vi "Holzworth.vi"(10 "Stop Point":string, 11 "Holzworth":refnum<visa-resource-name>="COM9") -> (2 "Amplitudes":string[](array[string]), 3 "Frequencies":string[](array[string]))   [LabVIEW 2023]
uses:
  <vilib>/regexp/Match Regular Expression.xnode
panel:
  out "read buffer 9":string
  out "read buffer 8":string
  out "read buffer 7":string
  out "read buffer 6":string
  out "read buffer 5":string
  out "read buffer 4":string
  out "read buffer 2":string
  out "points":dbl
  out "Comma Count":i32
  out "String 2":string
  out "String":string
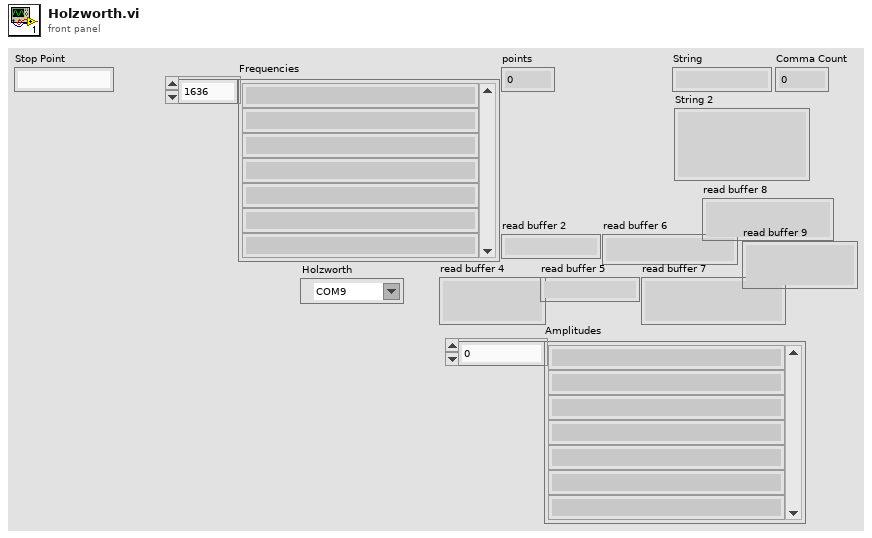
[diagram p1: front panel]
diagram:
  n1 = VISA Open(VISA resource name="Holzworth") -> (VISA resource name=w87:refnum<visa-resource-name>, error out=w84:errorcluster)  [unwired: 4 in]
  n2 = VISA Set I/O Buffer Size(VISA resource name=w87, size (4096)=u32 30000, error in (no error)=w84) -> (VISA resource name out=w86:refnum<visa-resource-name>, error out=w85:errorcluster)  [unwired: 1 in]
  n3 = VISA Flush I/O Buffer(VISA resource name=w86, error in (no error)=w85) -> (VISA resource name out=w4:refnum<visa-resource-name>, error out=w3:errorcluster)  [unwired: 1 in]
  n4 = Concatenate Strings("*RST" ("write buffer"), "\r") -> (w158:string)
  n5 = VISA Write(VISA resource name=w4, write buffer=w158, error in (no error)=w3) -> (VISA resource name out=w92:refnum<visa-resource-name>, error out=w90:errorcluster)  [unwired: 1 out]
  n6 = flat-sequence {
    tunnel: w92 -> [w163]
    tunnel: [w163] -> w91
    tunnel: w90 -> [w162]
    tunnel: [w162] -> w89
    tunnel: [w168] -> w48
    tunnel: [w169] -> w47
    tunnel: w91 -> [w167]
    tunnel: w89 -> [w166]
    frame #0 {
      n7 = Wait (ms)(milliseconds to wait=u32 2000) -> ()  [unwired: 1 out]
    }
    frame #1 {
      n8 = VISA Read(VISA resource name=w167, byte count=u32 256, error in (no error)=w166) -> (VISA resource name out=w168:refnum<visa-resource-name>, read buffer=→"read buffer 2":string, error out=w169:errorcluster)  [unwired: 1 out]
    }
  }
  n9 = Concatenate Strings(":SENS:PN:MEAS:TYPE:ABSOLUTE" ("write buffer"), "\r") -> (w58:string)
  n10 = VISA Write(VISA resource name=w48, write buffer=w58, error in (no error)=w47) -> (VISA resource name out=w60:refnum<visa-resource-name>, error out=w59:errorcluster)  [unwired: 1 out]
  n11 = flat-sequence {
    tunnel: w60 -> [w172]
    tunnel: [w172] -> w62
    tunnel: w59 -> [w171]
    tunnel: [w171] -> w61
    tunnel: [w177] -> w50
    tunnel: [w178] -> w49
    tunnel: w62 -> [w176]
    tunnel: w61 -> [w175]
    frame #0 {
      n12 = Wait (ms)(milliseconds to wait=u32 2000) -> ()  [unwired: 1 out]
    }
    frame #1 {
      n13 = VISA Read(VISA resource name=w176, byte count=u32 256, error in (no error)=w175) -> (VISA resource name out=w177:refnum<visa-resource-name>, read buffer=→"read buffer 4":string, error out=w178:errorcluster)  [unwired: 1 out]
    }
  }
  n14 = Concatenate Strings(":SENS:PN:MODE:SINGLE" ("write buffer"), "\r") -> (w51:string)
  n15 = VISA Write(VISA resource name=w50, write buffer=w51, error in (no error)=w49) -> (VISA resource name out=w53:refnum<visa-resource-name>, error out=w52:errorcluster)  [unwired: 1 out]
  n16 = flat-sequence {
    tunnel: w53 -> [w181]
    tunnel: [w181] -> w57
    tunnel: w52 -> [w180]
    tunnel: [w180] -> w56
    tunnel: [w187] -> w38
    tunnel: w57 -> [w186]
    tunnel: w56 -> [w185]
    tunnel: [w184] -> w39
    frame #0 {
      n17 = Wait (ms)(milliseconds to wait=u32 2000) -> ()  [unwired: 1 out]
    }
    frame #1 {
      n18 = VISA Read(VISA resource name=w186, byte count=u32 256, error in (no error)=w185) -> (VISA resource name out=w184:refnum<visa-resource-name>, read buffer=→"read buffer 5":string, error out=w187:errorcluster)  [unwired: 1 out]
    }
  }
  n19 = Concatenate Strings(":SENS:PN:CORR:COUN:1000" ("write buffer"), "\r") -> (w40:string)
  n20 = VISA Write(VISA resource name=w39, write buffer=w40, error in (no error)=w38) -> (VISA resource name out=w42:refnum<visa-resource-name>, error out=w41:errorcluster)  [unwired: 1 out]
  n21 = flat-sequence {
    tunnel: w42 -> [w190]
    tunnel: [w190] -> w44
    tunnel: w41 -> [w189]
    tunnel: [w189] -> w43
    tunnel: [w196] -> w29
    tunnel: w44 -> [w195]
    tunnel: w43 -> [w194]
    tunnel: [w193] -> w30
    frame #0 {
      n22 = Wait (ms)(milliseconds to wait=u32 2000) -> ()  [unwired: 1 out]
    }
    frame #1 {
      n23 = VISA Read(VISA resource name=w195, byte count=u32 256, error in (no error)=w194) -> (VISA resource name out=w196:refnum<visa-resource-name>, read buffer=→"read buffer 6":string, error out=w193:errorcluster)  [unwired: 1 out]
    }
  }
  n24 = Concatenate Strings(":SENS:PN:VCO:TRUE" ("write buffer"), "\r") -> (w32:string)
  n25 = VISA Write(VISA resource name=w29, write buffer=w32, error in (no error)=w30) -> (VISA resource name out=w34:refnum<visa-resource-name>, error out=w33:errorcluster)  [unwired: 1 out]
  n26 = flat-sequence {
    tunnel: w34 -> [w199]
    tunnel: [w199] -> w37
    tunnel: w33 -> [w198]
    tunnel: [w198] -> w36
    tunnel: [w205] -> w21
    tunnel: w37 -> [w204]
    tunnel: w36 -> [w203]
    tunnel: [w202] -> w20
    frame #0 {
      n27 = Wait (ms)(milliseconds to wait=u32 2000) -> ()  [unwired: 1 out]
    }
    frame #1 {
      n28 = VISA Read(VISA resource name=w204, byte count=u32 256, error in (no error)=w203) -> (VISA resource name out=w205:refnum<visa-resource-name>, read buffer=→"read buffer 7":string, error out=w202:errorcluster)  [unwired: 1 out]
    }
  }
  n29 = Concatenate Strings(":SENS:PN:LO:STATUS:INT" ("write buffer"), "\r") -> (w22:string)
  n30 = VISA Write(VISA resource name=w21, write buffer=w22, error in (no error)=w20) -> (VISA resource name out=w24:refnum<visa-resource-name>, error out=w23:errorcluster)  [unwired: 1 out]
  n31 = flat-sequence {
    tunnel: w24 -> [w208]
    tunnel: [w208] -> w26
    tunnel: w23 -> [w207]
    tunnel: [w207] -> w25
    tunnel: [w214] -> w11
    tunnel: w26 -> [w213]
    tunnel: w25 -> [w212]
    tunnel: [w211] -> w12
    frame #0 {
      n32 = Wait (ms)(milliseconds to wait=u32 2000) -> ()  [unwired: 1 out]
    }
    frame #1 {
      n33 = VISA Read(VISA resource name=w213, byte count=u32 256, error in (no error)=w212) -> (VISA resource name out=w211:refnum<visa-resource-name>, read buffer=→"read buffer 8":string, error out=w214:errorcluster)  [unwired: 1 out]
    }
  }
  n34 = Concatenate Strings(":SENS:PN:DATA:TYPE:CROSS" ("write buffer"), "\r") -> (w14:string)
  n35 = VISA Write(VISA resource name=w12, write buffer=w14, error in (no error)=w11) -> (VISA resource name out=w16:refnum<visa-resource-name>, error out=w15:errorcluster)  [unwired: 1 out]
  n36 = flat-sequence {
    tunnel: w16 -> [w217]
    tunnel: [w217] -> w19
    tunnel: w15 -> [w216]
    tunnel: [w216] -> w18
    tunnel: [w223] -> w7
    tunnel: w19 -> [w222]
    tunnel: w18 -> [w221]
    tunnel: [w220] -> w8
    frame #0 {
      n37 = Wait (ms)(milliseconds to wait=u32 2000) -> ()  [unwired: 1 out]
    }
    frame #1 {
      n38 = VISA Read(VISA resource name=w222, byte count=u32 256, error in (no error)=w221) -> (VISA resource name out=w220:refnum<visa-resource-name>, read buffer=→"read buffer 9":string, error out=w223:errorcluster)  [unwired: 1 out]
    }
  }
  n39 = Concatenate Strings(":SENS:PN:FREQ:STAR:1Hz" ("write buffer"), "\r") -> (w155:string)
  n40 = VISA Write(VISA resource name=w8, write buffer=w155, error in (no error)=w7) -> (VISA resource name out=w122:refnum<visa-resource-name>, error out=w123:errorcluster)  [unwired: 1 out]
  n41 = flat-sequence {
    tunnel: w123 -> [w229]
    tunnel: w122 -> [w227]
    tunnel: [w226] -> w105
    tunnel: [w225] -> w104
    tunnel: [w231] -> w68
    tunnel: w105 -> [w231]
    tunnel: w104 -> [w230]
    tunnel: [w230] -> w69
    frame #0 {
      n42 = VISA Read(VISA resource name=w227, byte count=u32 256, error in (no error)=w229) -> (VISA resource name out=w226:refnum<visa-resource-name>, error out=w225:errorcluster)  [unwired: 2 out]
    }
    frame #1 {
      n43 = Wait (ms)(milliseconds to wait=u32 5000) -> ()  [unwired: 1 out]
    }
  }
  n44 = Concatenate Strings(":SENS:PN:FREQ:STOP:" ("write buffer"), "Stop Point", "\r") -> (w67:string)
  n45 = VISA Write(VISA resource name=w68, write buffer=w67, error in (no error)=w69) -> (VISA resource name out=w70:refnum<visa-resource-name>, error out=w71:errorcluster)  [unwired: 1 out]
  n46 = flat-sequence {
    tunnel: w71 -> [w237]
    tunnel: w70 -> [w235]
    tunnel: [w234] -> w73
    tunnel: [w233] -> w72
    tunnel: [w239] -> w1
    tunnel: w73 -> [w239]
    tunnel: w72 -> [w238]
    tunnel: [w238] -> w2
    frame #0 {
      n47 = VISA Read(VISA resource name=w235, byte count=u32 256, error in (no error)=w237) -> (VISA resource name out=w234:refnum<visa-resource-name>, error out=w233:errorcluster)  [unwired: 2 out]
    }
    frame #1 {
      n48 = Wait (ms)(milliseconds to wait=u32 5000) -> ()  [unwired: 1 out]
    }
  }
  n49 = while {
    shift-right: [w255] -> w9
    shift-left: w1 -> [w243]
    shift-right: [w254] -> w10
    shift-left: w2 -> [w242]
    stop <- w248 stop-if-true
    n50 = Concatenate Strings(":STAT:OPER:COND?" ("write buffer"), "\r") -> (w245:string)
    n51 = VISA Write(VISA resource name=w243, write buffer=w245, error in (no error)=w242) -> (VISA resource name out=w244:refnum<visa-resource-name>, error out=w241:errorcluster)  [unwired: 1 out]
    n52 = VISA Read(VISA resource name=w244, byte count=u32 256, error in (no error)=w241) -> (VISA resource name out=w255:refnum<visa-resource-name>, read buffer=w253:string, error out=w254:errorcluster)  [unwired: 1 out]
    n53 = xnode "Match Regular Expression"("input string"=w253, "regular expression"="Instrument Ready") -> ("offset past match"=w251:i32)  [unwired: 4 in, 4 out]
    n54 = Not Equal?(x=w251, y=-1) -> (x != y?=w248:bool)
  }
  n55 = Concatenate Strings(":SENS:PN:SAMPLES:COUN:512" ("write buffer"), "\r") -> (w152:string)
  n56 = VISA Write(VISA resource name=w9, write buffer=w152, error in (no error)=w10) -> (VISA resource name out=w129:refnum<visa-resource-name>, error out=w131:errorcluster)  [unwired: 1 out]
  n57 = flat-sequence {
    tunnel: w131 -> [w377]
    tunnel: u32 256 ("byte count") -> [w376]
    tunnel: w129 -> [w375]
    tunnel: [w374] -> w109
    tunnel: [w373] -> w107
    tunnel: w109 -> [w379]
    tunnel: [w379] -> w108
    tunnel: [w378] -> w106
    tunnel: w107 -> [w378]
    frame #0 {
      n58 = VISA Read(VISA resource name=w375, byte count=w376, error in (no error)=w377) -> (VISA resource name out=w374:refnum<visa-resource-name>, error out=w373:errorcluster)  [unwired: 2 out]
    }
    frame #1 {
      n59 = Wait (ms)(milliseconds to wait=u32 5000) -> ()  [unwired: 1 out]
    }
  }
  n60 = while {
    shift-right: [w382] -> _
    shift-left: w108 -> [w385]
    shift-right: [w381] -> _
    shift-left: w106 -> [w384]
    tunnel: [w382] -> w143
    tunnel: [w381] -> w142
    stop <- w390 stop-if-true
    n61 = Concatenate Strings(":STAT:OPER:COND?" ("write buffer"), "\r") -> (w387:string)
    n62 = VISA Write(VISA resource name=w385, write buffer=w387, error in (no error)=w384) -> (VISA resource name out=w386:refnum<visa-resource-name>, error out=w383:errorcluster)  [unwired: 1 out]
    n63 = VISA Read(VISA resource name=w386, byte count=u32 256, error in (no error)=w383) -> (VISA resource name out=w382:refnum<visa-resource-name>, read buffer=w395:string, error out=w381:errorcluster)  [unwired: 1 out]
    n64 = xnode "Match Regular Expression"("input string"=w395, "regular expression"="Instrument Ready") -> ("offset past match"=w393:i32)  [unwired: 4 in, 4 out]
    n65 = Not Equal?(x=w393, y=-1) -> (x != y?=w390:bool)
  }
  n66 = Concatenate Strings(":INIT:PN:CAL" ("write buffer"), "\r") -> (w149:string)
  n67 = VISA Write(VISA resource name=w143, write buffer=w149, error in (no error)=w142) -> (VISA resource name out=w126:refnum<visa-resource-name>, error out=w128:errorcluster)  [unwired: 1 out]
  n68 = flat-sequence {
    tunnel: w128 -> [w517]
    tunnel: u32 256 ("byte count") -> [w516]
    tunnel: w126 -> [w515]
    tunnel: [w514] -> w113
    tunnel: [w513] -> w111
    tunnel: [w519] -> w112
    tunnel: w113 -> [w519]
    tunnel: [w518] -> w110
    tunnel: w111 -> [w518]
    frame #0 {
      n69 = VISA Read(VISA resource name=w515, byte count=w516, error in (no error)=w517) -> (VISA resource name out=w514:refnum<visa-resource-name>, error out=w513:errorcluster)  [unwired: 2 out]
    }
    frame #1 {
      n70 = Wait (ms)(milliseconds to wait=u32 5000) -> ()  [unwired: 1 out]
    }
  }
  n71 = while {
    shift-right: [w535] -> w6
    shift-left: w112 -> [w523]
    shift-right: [w534] -> w5
    shift-left: w110 -> [w522]
    stop <- w528 stop-if-true
    n72 = Concatenate Strings(":STAT:OPER:COND?" ("write buffer"), "\r") -> (w525:string)
    n73 = VISA Write(VISA resource name=w523, write buffer=w525, error in (no error)=w522) -> (VISA resource name out=w524:refnum<visa-resource-name>, error out=w521:errorcluster)  [unwired: 1 out]
    n74 = VISA Read(VISA resource name=w524, byte count=u32 256, error in (no error)=w521) -> (VISA resource name out=w535:refnum<visa-resource-name>, read buffer=w533:string, error out=w534:errorcluster)  [unwired: 1 out]
    n75 = xnode "Match Regular Expression"("input string"=w533, "regular expression"="Instrument Ready") -> ("offset past match"=w531:i32)  [unwired: 4 in, 4 out]
    n76 = Not Equal?(x=w531, y=-1) -> (x != y?=w528:bool)
  }
  n77 = VISA Clear(VISA resource name=w6, error in (no error)=w5) -> (VISA resource name out=w145:refnum<visa-resource-name>, error out=w144:errorcluster)
  n78 = Concatenate Strings(":INIT:PN:IMM" ("write buffer"), "\r") -> (w146:string)
  n79 = VISA Write(VISA resource name=w145, write buffer=w146, error in (no error)=w144) -> (VISA resource name out=w124:refnum<visa-resource-name>, error out=w125:errorcluster)  [unwired: 1 out]
  n80 = flat-sequence {
    tunnel: w125 -> [w657]
    tunnel: w124 -> [w655]
    tunnel: [w654] -> w121
    tunnel: [w653] -> w119
    tunnel: [w659] -> w120
    tunnel: w121 -> [w659]
    tunnel: [w658] -> w118
    tunnel: w119 -> [w658]
    frame #0 {
      n81 = VISA Read(VISA resource name=w655, byte count=u32 256, error in (no error)=w657) -> (VISA resource name out=w654:refnum<visa-resource-name>, error out=w653:errorcluster)  [unwired: 2 out]
    }
    frame #1 {
      n82 = Wait (ms)(milliseconds to wait=u32 10000) -> ()  [unwired: 1 out]
    }
  }
  n83 = while {
    shift-right: [w675] -> w96
    shift-left: w120 -> [w663]
    shift-right: [w674] -> w95
    shift-left: w118 -> [w662]
    stop <- w668 stop-if-true
    n84 = Concatenate Strings(":STAT:OPER:COND?" ("write buffer"), "\r") -> (w665:string)
    n85 = VISA Write(VISA resource name=w663, write buffer=w665, error in (no error)=w662) -> (VISA resource name out=w664:refnum<visa-resource-name>, error out=w661:errorcluster)  [unwired: 1 out]
    n86 = VISA Read(VISA resource name=w664, byte count=u32 256, error in (no error)=w661) -> (VISA resource name out=w675:refnum<visa-resource-name>, read buffer=w673:string, error out=w674:errorcluster)  [unwired: 1 out]
    n87 = xnode "Match Regular Expression"("input string"=w673, "regular expression"="Instrument Ready") -> ("offset past match"=w671:i32)  [unwired: 4 in, 4 out]
    n88 = Not Equal?(x=w671, y=-1) -> (x != y?=w668:bool)
  }
  n89 = Concatenate Strings(":SENS:PN:SWE:POIN? " ("write buffer"), "\r") -> (w97:string)
  n90 = VISA Write(VISA resource name=w96, write buffer=w97, error in (no error)=w95) -> (VISA resource name out=w99:refnum<visa-resource-name>, error out=w98:errorcluster)  [unwired: 1 out]
  n91 = flat-sequence {
    tunnel: [w795] -> w101
    tunnel: [w794] -> w100
    tunnel: w98 -> [w796]
    tunnel: w99 -> [w797]
    tunnel: [w793] -> w75
    tunnel: w101 -> [w801]
    tunnel: w100 -> [w802]
    tunnel: [w802] -> w94
    tunnel: [w801] -> w93
    tunnel: w75 -> [w800]
    frame #0 {
      n92 = VISA Read(VISA resource name=w797, byte count=u32 256, error in (no error)=w796) -> (VISA resource name out=w794:refnum<visa-resource-name>, read buffer=w793:string, error out=w795:errorcluster)  [unwired: 1 out]
    }
    frame #1 {
      n93 = Fract/Exp String To Number(string=w800) -> (number=→"points":dbl)  [unwired: 3 in, 1 out]
      n94 = Wait (ms)(milliseconds to wait=u32 5000) -> ()  [unwired: 1 out]
    }
  }
  n95 = Concatenate Strings(":CALC:PN:DATA:XDAT?" ("write buffer"), "\r") -> (w138:string)
  n96 = VISA Write(VISA resource name=w94, write buffer=w138, error in (no error)=w93) -> (VISA resource name out=w117:refnum<visa-resource-name>, error out=w116:errorcluster)  [unwired: 1 out]
  n97 = while {
    shift-right: [w814] -> w77
    shift-left: w117 -> [w817]
    shift-right: [w815] -> w76
    shift-left: w116 -> [w816]
    shift-right: [w810] -> w88
    shift-left: "" -> [w811]
    stop <- w806 stop-if-true
    n98 = flat-sequence {
      tunnel: w817 -> [w824]
      tunnel: [w824] -> w821
      tunnel: w816 -> [w823]
      tunnel: [w823] -> w820
      tunnel: w821 -> [w830]
      tunnel: w820 -> [w829]
      tunnel: [w828] -> w819
      tunnel: [w827] -> w818
      tunnel: [w826] -> w804
      tunnel: w819 -> [w834]
      tunnel: w818 -> [w833]
      tunnel: [w834] -> w813
      tunnel: [w833] -> w812
      tunnel: [w832] -> w805
      tunnel: w804 -> [w832]
      tunnel: w813 -> [w840]
      tunnel: w812 -> [w839]
      tunnel: w811 -> [w838]
      tunnel: [w840] -> w809
      tunnel: [w839] -> w808
      tunnel: [w837] -> w807
      tunnel: w805 -> [w836]
      tunnel: [w969] -> w810
      tunnel: [w970] -> w814
      tunnel: [w971] -> w815
      tunnel: w809 -> [w971]
      tunnel: w808 -> [w970]
      tunnel: w807 -> [w969]
      tunnel: [w967] -> w806
      frame #0 {
        n99 = local write "Comma Count"(0 ("Comma Count")) -> ()
        n100 = Wait (ms)(milliseconds to wait=u32 1000) -> ()  [unwired: 1 out]
      }
      frame #1 {
        n101 = VISA Read(VISA resource name=w830, byte count=u32 8192, error in (no error)=w829) -> (VISA resource name out=w827:refnum<visa-resource-name>, read buffer=w826:string, error out=w828:errorcluster)  [unwired: 1 out]
      }
      frame #2 {
        n102 = Wait (ms)(milliseconds to wait=u32 1000) -> ()  [unwired: 1 out]
      }
      frame #3 {
        n103 = Concatenate Strings(w838, w836) -> (w837:string)
        n104 = while {
          shift-right: [w843] -> _
          shift-left: w837 -> [w845]
          i -> [w841]
          stop <- w842 stop-if-true
          n105 = xnode "Match Regular Expression"("input string"=w845, "regular expression"=",") -> ("after match"=w843:string, "offset past match"=w847:i32)  [unwired: 4 in, 3 out]
          n106 = Equal?(x=w847, y=-1) -> (x = y?=w842:bool)
          "Comma Count" <- w841
        }
      }
      frame #4 {
        n107 = local read "Comma Count"() -> (w968:i32)
        n108 = local read "points"() -> (w966:dbl)
        n109 = Decrement(x=w966) -> (x-1=w965:dbl)
        n110 = Equal?(x=w968, y=w965) -> (x = y?=w967:bool)
      }
    }
  }
  "String" <- w88
  n111 = Concatenate Strings(":CALC:PN:DATA:FDAT?" ("write buffer"), "\r") -> (w134:string)
  n112 = VISA Write(VISA resource name=w77, write buffer=w134, error in (no error)=w76) -> (VISA resource name out=w115:refnum<visa-resource-name>, error out=w114:errorcluster)  [unwired: 1 out]
  n113 = call <vilib>:"Delimited String to 1D String Array.vi"("delimiter"=",", "delimited string"=w88) -> ("string array"=→"Frequencies":string[])  [unwired: 9 in]
  n114 = while {
    tunnel: w115 -> [w985]
    tunnel: w114 -> [w984]
    shift-right: [w974] -> w80
    shift-left: "" -> [w979]
    tunnel: [w983] -> w79
    tunnel: [w982] -> w78
    stop <- w976 stop-if-true
    n115 = flat-sequence {
      tunnel: w985 -> [w992]
      tunnel: [w992] -> w989
      tunnel: w984 -> [w991]
      tunnel: [w991] -> w988
      tunnel: w989 -> [w998]
      tunnel: w988 -> [w997]
      tunnel: [w996] -> w987
      tunnel: [w995] -> w986
      tunnel: [w994] -> w972
      tunnel: w987 -> [w1002]
      tunnel: w986 -> [w1001]
      tunnel: [w1002] -> w981
      tunnel: [w1001] -> w980
      tunnel: [w1000] -> w973
      tunnel: w972 -> [w1000]
      tunnel: w980 -> [w1007]
      tunnel: w981 -> [w1008]
      tunnel: w979 -> [w1006]
      tunnel: [w1008] -> w978
      tunnel: [w1007] -> w977
      tunnel: [w1005] -> w975
      tunnel: w973 -> [w1004]
      tunnel: [w1138] -> w982
      tunnel: [w1139] -> w983
      tunnel: w978 -> [w1139]
      tunnel: w977 -> [w1138]
      tunnel: [w1136] -> w976
      tunnel: w975 -> [w1135]
      tunnel: [w1135] -> w974
      frame #0 {
        n116 = local write "Comma Count"(0 ("Comma Count")) -> ()
        n117 = Wait (ms)(milliseconds to wait=u32 1000) -> ()  [unwired: 1 out]
      }
      frame #1 {
        n118 = VISA Read(VISA resource name=w998, byte count=u32 8192, error in (no error)=w997) -> (VISA resource name out=w995:refnum<visa-resource-name>, read buffer=w994:string, error out=w996:errorcluster)  [unwired: 1 out]
      }
      frame #2 {
        n119 = Wait (ms)(milliseconds to wait=u32 1000) -> ()  [unwired: 1 out]
      }
      frame #3 {
        n120 = Concatenate Strings(w1006, w1004) -> (w1005:string)
        n121 = while {
          shift-right: [w1011] -> _
          shift-left: w1005 -> [w1013]
          i -> [w1009]
          stop <- w1010 stop-if-true
          n122 = xnode "Match Regular Expression"("input string"=w1013, "regular expression"=",") -> ("after match"=w1011:string, "offset past match"=w1015:i32)  [unwired: 4 in, 3 out]
          n123 = local write "Comma Count"(w1009) -> ()
          n124 = Equal?(x=w1015, y=-1) -> (x = y?=w1010:bool)
        }
      }
      frame #4 {
        n125 = local read "Comma Count"() -> (w1137:i32)
        n126 = local read "points"() -> (w1133:dbl)
        n127 = Decrement(x=w1133) -> (x-1=w1134:dbl)
        n128 = Equal?(x=w1137, y=w1134) -> (x = y?=w1136:bool)
      }
    }
  }
  "String 2" <- w80
  n129 = VISA Close(VISA resource name=w78, error in (no error)=w79) -> ()  [unwired: 1 out]
  n130 = call <vilib>:"Delimited String to 1D String Array.vi"("delimiter"=",", "delimited string"=w80) -> ("string array"=→"Amplitudes":string[])  [unwired: 9 in]
